vi "varXNode_Mutate_1_0_0_1.vi"(8 "error in (no error)":errorcluster, 10 "Version":T1, 11 "Old State":variant) -> (0 "error out":errorcluster, 1 "Replies out":string[](array[string]), 2 "Version Out":T1, 3 "New State":variant)   [LabVIEW 2020, in "varXNode.xnode"]
uses:
  <vilib>/variable/varXNode.llb/varXNode.xnode
  <vilib>/XNodeSupport/XNodeVersion.ctl
  <vilib>/XNodeSupport/XNodeUShort.ctl
  <vilib>/variable/varXNode.llb/varXNode_old_1_0_0_0.ctl
  <vilib>/variable/varXNode.llb/varXNode_old_1_0_0_2.ctl
  <vilib>/XNodeSupport/NI_XNodeSupport.lvlib
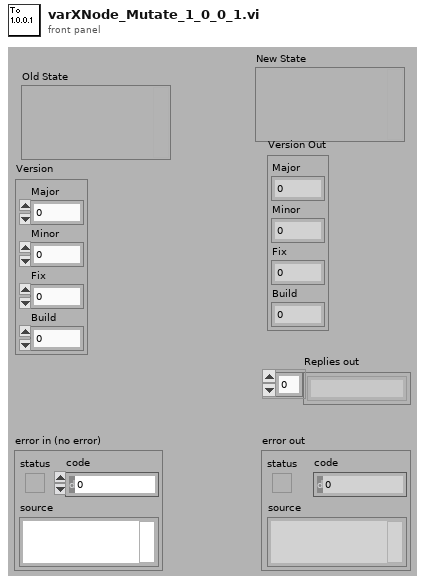
[diagram p1: front panel]
types:
  T1 = typedef "NI_XNodeSupport.lvlib/XNodeVersion.ctl" = cluster{"Major":T2, "Minor":T2, "Fix":T2, "Build":T2}
  T2 = typedef "NI_XNodeSupport.lvlib/XNodeUShort.ctl" = u16
  T3 = typedef "varXNode.xnode/varXNode_old_1_0_0_0.ctl" = cluster{"Write":bool, "VarHandle":u32, "VSItemID":string, "URL":string, "ShowTimestamp":bool, "RemoteTypeDesc":i16[], "CachedName":string, "CachedTypeDesc":i16[], "CachedFeaturePacks":string[]}
  T4 = typedef "varXNode.xnode/varXNode_old_1_0_0_2.ctl" = cluster{"Write":bool, "ShowTimestamp":bool, "CachedName":string, "CachedTypeDesc":i16[], "CachedFeaturePacks":string[], "Custom Rule":string, "ProjectPath":string}
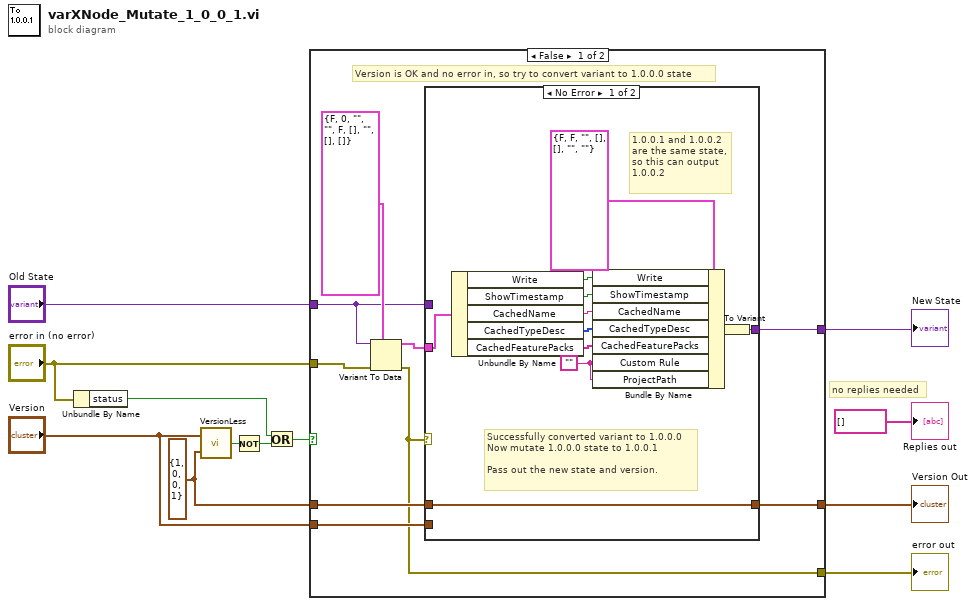
[diagram p0: block diagram]
diagram:
  w11 = T1 {"Major"=1, "Minor"=0, "Fix"=0, "Build"=1} ("y")
  # "no replies needed"
  n1 = Unbundle By Name("error in (no error)") -> ("status"=w3:bool)
  n2 = call <vilib>:"VersionLess.vi"("y"=w11, "x"="Version") -> ("x < y?"=w12:bool)
  n3 = Not(x=w12) -> (.not. x?=w2:bool)
  n4 = Or(x=w3, y=w2) -> (x .or. y?=w5:bool)
  n5 = case shown="False" w5 {
    tunnel: w11 -> [w21 _]
    tunnel: [w18 w37] -> w10
    tunnel: "Old State" -> [w17 w37]
    tunnel: [w16 w36] -> w8
    tunnel: "Version" -> [w15 w36]
    tunnel: [w14 w35] -> w6
    tunnel: "error in (no error)" -> [w13 w35]
    frame False {
      # "Version is OK and no error in, so try to convert variant to 1.0.0.0 state"
      n6 = Variant To Data(error in=w13, type=T3 {"Write"=FALSE, "VarHandle"=0, "VSItemID"="", "URL"="", "ShowTimestamp"=FALSE, "RemoteTypeDesc"=[], "CachedName"="", "CachedTypeDesc"=[], "CachedFeaturePacks"=[]} ("State"), Variant=w17) -> (data=w19:T3, error out=w14:errorcluster)
      n7 = case shown="No Error" w14 {
        tunnel: w21 -> [w28 _]
        tunnel: w19 -> [w32 _]
        tunnel: [w29 w34] -> w18
        tunnel: w17 -> [_ w34]
        tunnel: [w28 w33] -> w16
        tunnel: w15 -> [_ w33]
        frame No Error {
          w22 = ""
          # "1.0.0.1 and 1.0.0.2\nare the same state,\nso this can output\n1.0.0.2"
          # "Successfully converted variant to 1.0.0.0\nNow mutate 1.0.0.0 state to 1.0.0.1\n\nPass out the new state and version."
          n8 = Unbundle By Name(w32) -> ("Write"=w27:bool, "ShowTimestamp"=w26:bool, "CachedName"=w25:string, "CachedTypeDesc"=w24:i16[], "CachedFeaturePacks"=w23:string[])
          n9 = Bundle By Name(cluster=T4 {"Write"=FALSE, "ShowTimestamp"=FALSE, "CachedName"="", "CachedTypeDesc"=[], "CachedFeaturePacks"=[], "Custom Rule"="", "ProjectPath"=""} ("State"), "Write"=w27, "ShowTimestamp"=w26, "CachedName"=w25, "CachedTypeDesc"=w24, "CachedFeaturePacks"=w23, "Custom Rule"=w22, "ProjectPath"=w22) -> (w30:T4)
          n10 = To Variant(anything=w30) -> (Variant=w29:variant)
        }
        frame Error {
          # "Couldn't convert variant to 1.0.0.0 state\nPass the input values out"
        }
      }
    }
    frame True {
      # "Either there was an error in,\nor the version is not less than 1.0.0.1.\nPass input values out."
    }
  }
  "New State" <- w10
  "Version Out" <- w8
  "error out" <- w6
  "Replies out" <- string[] [] ("Replies out")
